vi "Example - Continuous Acquisition v1.0.vi"() -> ()   [LabVIEW 2015, in "Monitoring_receiver.lvlib"]
uses:
  Monitoring_receiver.lvlib
  <vilib>/userdefined/High Color/nirio_resource_hc.ctl
  <userlib>/SE-APP-Receiver/NI5772/7976R_v1/7976R_v1.lvclass
  <vilib>/measure/maspectr.llb/FFT Power Spectrum and PSD for 1 Chan (CDB).vi
  <vilib>/measure/NI_MAPro.lvlib
  <instrlib>/niScope/Configure/Trigger/niScope Configure Trigger Software.vi
  <instrlib>/niScope/Acquire/Fetch/niScope Fetch Cluster.vi
  <instrlib>/niScope/Controls/niScope acquisition type.ctl
panel:
  out "FPGA FIFO overflow":bool
  out "dma.overflow":bool
  out "output waveform":waveform(dbl)(graph)
  out "ddc.number.of.ch":u8
  in  "seconds to read":dbl=0.001 format="%#_13p"
  out "FAM Configured?":bool
  out "Fw Version":string="1.7.5"
  out "Host Loop iteration":i32=15181
  in  "Center Frequency (Hz)":dbl[](array[numeric])=[201100000.0] format="%_5p"
  in  "IQ Rate (Hz)":dbl[](array[numeric])=[1000000.0] format="%#_6p"
  out "Power Spectrum / PSD":cluster{"f0":dbl, "df":dbl, "magnitude":dbl[]}(graph)={"f0"=-500000.0, "df"=10.0, "magnitude"=array[100000 elements]}
  in  "Stop Button":bool
  in  "RIO0 Resource":T1="7976R"
  out "Update":bool=TRUE
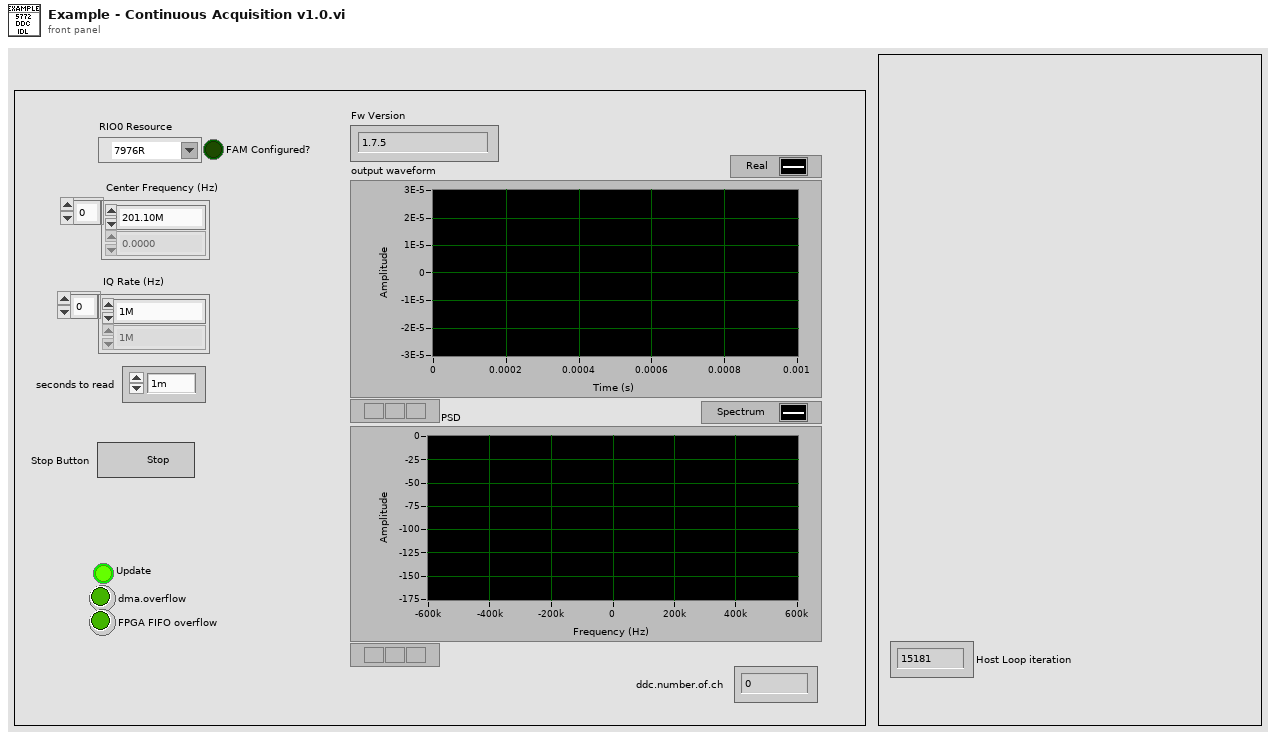
[diagram p1: front panel]
types:
  T1 = typedef "nirio_resource_hc.ctl" = tag
  T2 = enum16{"Normal mode", "TIS mode (CH0 only)", "TIS mode (CH1 only)"}
  T3 = enum8{"Internal Clock PLL Off", "Internal Clock PLL On (REF IN)", "External Clock (CLK_IN)", "Internal Clock PLL On (IoModSyncClk)"}
  T4 = cluster{"IQ Rate (Hz)":dbl[], "Freq Shift (Hz)":dbl[], "# of channels":u8, "Decimation factor":dbl[]}
  T5 = typedef "7976R_v1.lvclass/FPGA VI Reference_DDC_v1.8.ctl" = refnum<k20>
  T6 = cluster{"Bitfile Version":string, "FAM Configured":bool, "TIS Configured?":bool, "range (Vpp)":dbl, "Reference":T5}
  T7 = typedef "niScope acquisition type.ctl" = i32
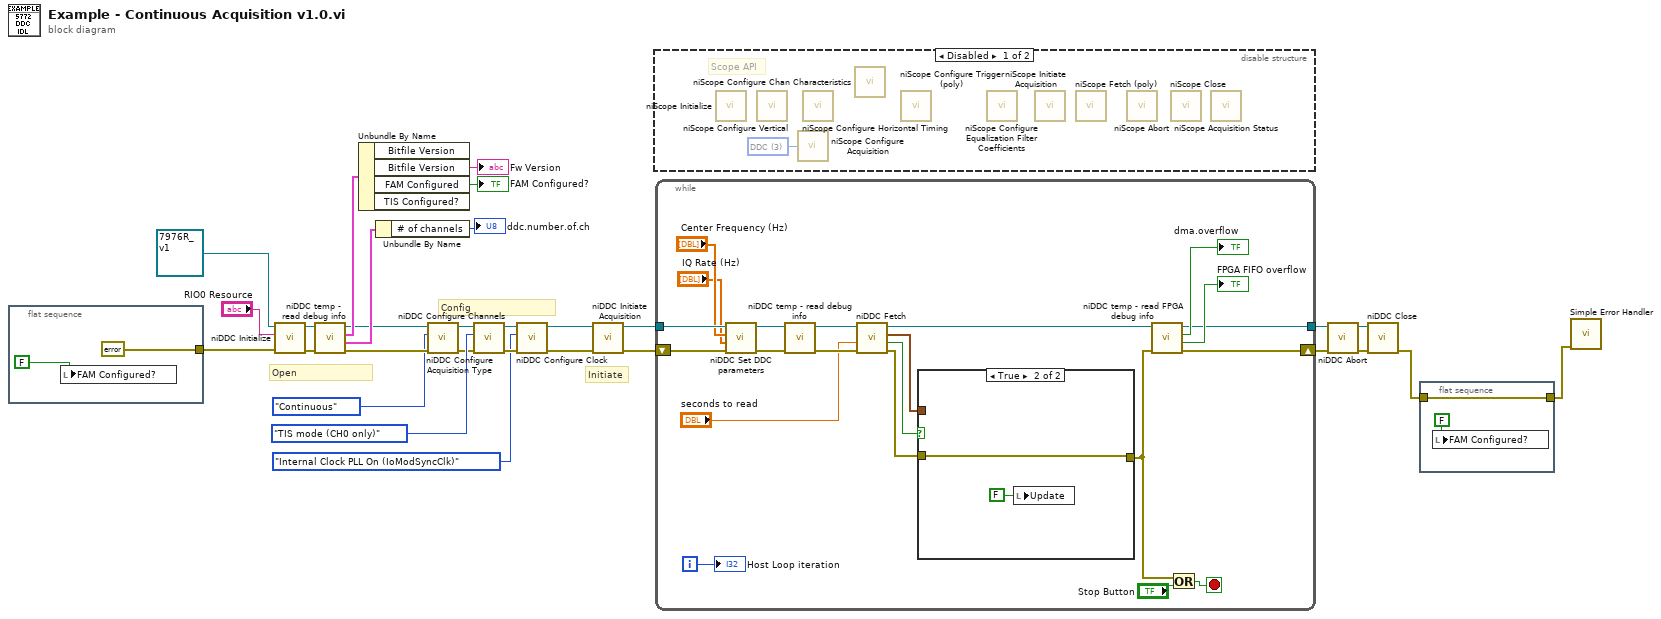
[diagram p0: block diagram]
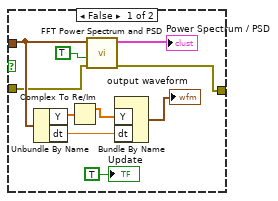
[diagram p2: hidden frame]
diagram:
  # "Open"
  # "Config"
  # "Initiate"
  n1 = flat-sequence {
    tunnel: [errorcluster {"status"=FALSE, "code"=0, "source"=""} ("error out")] -> w29
    frame #0 {
      n2 = local write "FAM Configured?"(FALSE ("Value")) -> ()
    }
  }
  n3 = call-dynamic "niDDC Initialize.vi"("error in (no error)"=w29, "RIO0 Resource"="RIO0 Resource", "Class in"=refnum<class "7976R_v1.lvclass"> refnum ("Monitoring_receiver.lvlib:7976R_v1.lvclass")) -> ("error out"=w20:errorcluster, "Class out"=w21:refnum<class "7976R_v1.lvclass">)  [unwired: 7 in]
  n4 = call-dynamic "niDDC temp - read debug info.vi"("error in (no error)"=w20, "Class in"=w21) -> ("error out"=w9:errorcluster, "DDC"=w12:T4, "FPGA"=w19:T6, "Class out"=w10:refnum<class "7976R_v1.lvclass">)  [unwired: 6 in]
  n5 = Unbundle By Name(w19) -> ("Bitfile Version"=→"Fw Version":string, "FAM Configured"=→"FAM Configured?":bool)  [unwired: 2 out]
  n6 = Unbundle By Name(w12) -> ("# of channels"=→"ddc.number.of.ch":u8)
  n7 = call-dynamic "niDDC Configure Acquisition Type.vi"("error in (no error)"=w9, "Type"=enum16{"Continuous", "Finite"}."Continuous", "Class in"=w10) -> ("error out"=w7:errorcluster, "Class out"=w8:refnum<class "7976R_v1.lvclass">)  [unwired: 7 in]
  n8 = call-dynamic "niDDC Configure Channels.vi"("error in (no error)"=w7, "mode"=T2."TIS mode (CH0 only)", "Class in"=w8) -> ("error out"=w23:errorcluster, "Class out"=w24:refnum<class "7976R_v1.lvclass">)  [unwired: 7 in]
  n9 = call-dynamic "niDDC Configure Clock.vi"("error in (no error)"=w23, "Clock Source"=T3."Internal Clock PLL On (IoModSyncClk)", "Class in"=w24) -> ("error out"=w15:errorcluster, "Class out"=w16:refnum<class "7976R_v1.lvclass">)  [unwired: 7 in]
  n10 = call-dynamic "niDDC Initiate Acquisition.vi"("error in (no error)"=w15, "Class in"=w16) -> ("error out"=w14:errorcluster, "Class out"=w13:refnum<class "7976R_v1.lvclass">)  [unwired: 8 in]
  n11 = disable-structure shown="Disabled" {
    frame Disabled {
      w32 = T7 3 items=["Normal"=0, "Flex Res"=1, "DDC"=3] ("acquisition Type")
      # "Scope API"
      n12 = call <instrlib>:"niScope Initialize.vi"() -> ()  [unwired: 14 in, 2 out]
      n13 = call <instrlib>:"niScope Configure Vertical.vi"() -> ()  [unwired: 14 in, 2 out]
      n14 = call <instrlib>:"niScope Configure Acquisition.vi"("acquisition Type"=w32) -> ()  [unwired: 13 in, 2 out]
      n15 = call <instrlib>:"niScope Configure Horizontal Timing.vi"() -> ()  [unwired: 14 in, 2 out]
      n16 = call <instrlib>:"niScope Configure Chan Characteristics.vi"() -> ()  [unwired: 14 in, 2 out]
      n17 = call-poly <instrlib>:"niScope Configure Trigger (poly).vi"() -> ()  [unwired: 14 in, 2 out]
      n18 = call <instrlib>:"niScope Configure Equalization Filter Coefficients.vi"() -> ()  [unwired: 10 in, 2 out]
      n19 = call <instrlib>:"niScope Initiate Acquisition.vi"() -> ()  [unwired: 14 in, 2 out]
      n20 = call-poly <instrlib>:"niScope Fetch (poly).vi"() -> ()  [unwired: 8 in, 4 out]
      n21 = call <instrlib>:"niScope Abort.vi"() -> ()  [unwired: 14 in, 2 out]
      n22 = call <instrlib>:"niScope Close.vi"() -> ()  [unwired: 15 in, 1 out]
      n23 = call <instrlib>:"niScope Acquisition Status.vi"() -> ()  [unwired: 13 in, 3 out]
    }
    frame Enabled {
    }
  }
  n24 = while {
    tunnel: w13 -> [w50]
    shift-right: [w37] -> w2
    shift-left: w14 -> [w49]
    tunnel: [w33] -> w4
    i -> [w51]
    stop <- w52 stop-if-true
    n25 = call-dynamic "niDDC Set DDC parameters.vi"("error in (no error)"=w49, "DDC IQ rates (Hz)"="IQ Rate (Hz)", "DDC Freq shift (Hz)"="Center Frequency (Hz)", "Class in"=w50) -> ("error out"=w45:errorcluster, "Class out"=w46:refnum<class "7976R_v1.lvclass">)  [unwired: 6 in]
    n26 = call-dynamic "niDDC temp - read debug info.vi"("error in (no error)"=w45, "Class in"=w46) -> ("error out"=w43:errorcluster, "Class out"=w44:refnum<class "7976R_v1.lvclass">)  [unwired: 6 in, 2 out]
    n27 = call-dynamic "niDDC Fetch.vi"("error in (no error)"=w43, "seconds to read (-1:all)"="seconds to read", "Class in"=w44) -> ("error out"=w42:errorcluster, "Timeout?"=w41:bool, "Complex wfm out"=w40:waveform(cdb), "Class out"=w38:refnum<class "7976R_v1.lvclass">)  [unwired: 5 in]
    n28 = case shown="True" w41 {
      tunnel: w42 -> [w56 w65]
      tunnel: w40 -> [w61 _]
      tunnel: [w55 w65] -> w36
      frame False {
        n29 = Unbundle By Name(w61) -> ("Y"=w58:cdb[], "dt"=w59:dbl)
        n30 = Complex To Re/Im(x + iy=w58) -> (x=w57:dbl[])  [unwired: 1 out]
        n31 = call-poly <vilib>:"FFT Power Spectrum and PSD.vi"("error in (no error)"=w56, "dB On (F)"=TRUE, "time signal"=w61) -> ("error out"=w55:errorcluster, "Power Spectrum / PSD"=→"Power Spectrum / PSD":cluster{"f0":dbl, "df":dbl, "magnitude":dbl[]})  [unwired: 5 in, 2 out]
        n32 = Bundle By Name("Y"=w57, "dt"=w59) -> (→"output waveform":waveform(dbl))  [unwired: 1 in]
        "Update" <- TRUE ("DDCRunnig")
      }
      frame True {
        n33 = local write "Update"(FALSE ("Update")) -> ()
      }
    }
    n34 = call-dynamic "niDDC temp - read FPGA debug info.vi"("error in (no error)"=w36, "Class in"=w38) -> ("error out"=w37:errorcluster, "FPGA FIFO overflow"=→"FPGA FIFO overflow":bool, "dma.overflow"=→"dma.overflow":bool, "Class out"=w33:refnum<class "7976R_v1.lvclass">)  [unwired: 5 in, 1 out]
    n35 = Or(x=w36, y="Stop Button") -> (x .or. y?=w52:bool)
    "Host Loop iteration" <- w51
  }
  n36 = call-dynamic "niDDC Abort.vi"("error in (no error)"=w2, "Class in"=w4) -> ("error out"=w1:errorcluster, "Class out"=w3:refnum<class "7976R_v1.lvclass">)  [unwired: 8 in]
  n37 = call-dynamic "niDDC Close.vi"("error in (no error)"=w1, "Class in"=w3) -> ("error out"=w5:errorcluster)  [unwired: 8 in, 1 out]
  n38 = flat-sequence {
    tunnel: w5 -> [w66]
    tunnel: [w66] -> w28
    frame #0 {
      n39 = local write "FAM Configured?"(FALSE ("Value")) -> ()
    }
  }
  n40 = call <vilib>:"Simple Error Handler.vi"("error in (no error)"=w28) -> ()  [unwired: 4 in, 5 out]
